vi "Release Queue Ref.vi"(8 "error in (no error)":errorcluster, 11 "Stack in":refnum<class "Stack.lvclass">) -> (0 "error out":errorcluster)   [LabVIEW 2012, in "Stack.lvlib" / "Stack.lvclass"]
doc: "Force releasing queue reference."
uses:
  Stack.lvclass
  Stack.lvclass/Stack.ctl
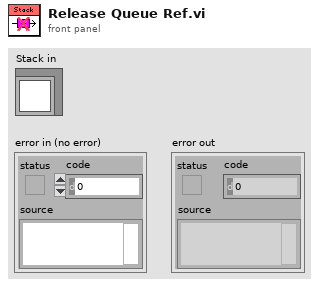
[diagram p1: front panel]
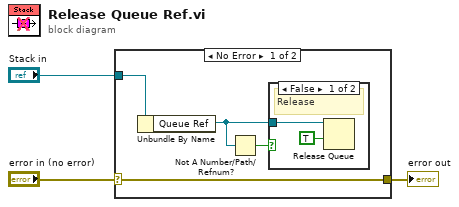
[diagram p0: block diagram]
diagram:
  n1 = case shown="No Error" "error in (no error)" {
    selector: "error in (no error)" -> [w7 w10]
    tunnel: [w7 w10] -> w2
    tunnel: "Stack in" -> [w6 _]
    frame No Error {
      n2 = Unbundle By Name(w6) -> ("Queue Ref"=w5:refnum<queue>)
      n3 = Not A Number/Path/Refnum?(number/path/refnum=w5) -> (NaN/Path/Refnum?=w4:bool)
      n4 = case shown="False" w4 {
        tunnel: w5 -> [w9 _]
        frame False {
          # "Release"
          n5 = Release Queue(queue=w9, force destroy? (F)=TRUE) -> ()  [unwired: 1 in, 3 out]
        }
        frame True {
        }
      }
    }
    frame Error {
    }
  }
  "error out" <- w2
